vi "WPI_CounterConfigureTimer.vi"(8 "error in (no error)":errorcluster, 9 "Number Samples to Average":u8=1 min=1 max=128, 10 "MaxPeriod (sec)":dbl=0.05, 11 "CounterDevRef in":T1) -> (0 "error out":errorcluster, 3 "CounterDevRef out":T1)   [LabVIEW 2017]
doc: "Configures the timer on the counter. Use this VI to specify the maximum time between pulses that can elapse before the application considers the counter stopped and to specify the number of samples of the timer to average when calculating the period. Use the Get VI to determine whether the counter is stopped.\n\nThis software is licensed. Open the labview\\readme\\WPI Robotics Library Open Source License.txt file for more information."
uses:
  <vilib>/Rock Robotics/WPI/Counter/WPI_CounterDevRef.ctl
  <vilib>/Rock Robotics/SystemInterfaces/Counter/FPGA_CounterCtrSystemIndex.ctl
  <vilib>/Rock Robotics/SystemInterfaces/Counter/FPGA_CounterERRInvalidResource.vi
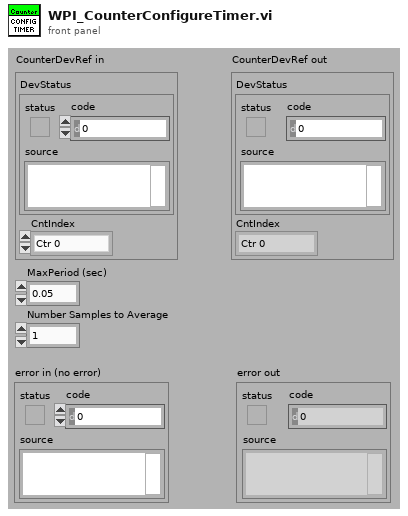
[diagram p1: front panel]
types:
  T1 = typedef "WPI_CounterDevRef.ctl" = cluster{"DevStatus":errorcluster, "CntIndex":T2}
  T2 = typedef "FPGA_CounterCtrSystemIndex.ctl" = enum8{"Ctr 0", "Ctr 1", "Ctr 2", "Ctr 3", "Ctr 4", "Ctr 5", "Ctr 6", "Ctr 7", "Invalid"}
  T3 = typedef "FPGA_CounterCtrDevRef.ctl" = cluster{"DevStatus":errorcluster, "CntIndex":T2}
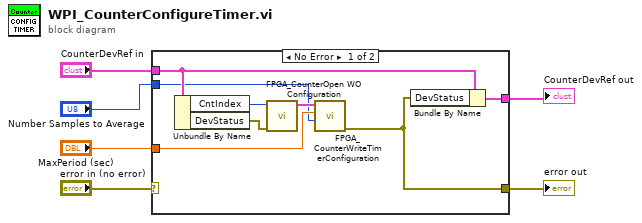
[diagram p0: block diagram]
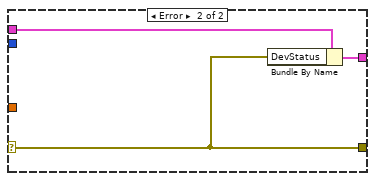
[diagram p2: hidden frame]
diagram:
  n1 = case shown="No Error" "error in (no error)" {
    selector: "error in (no error)" -> [_ w15]
    tunnel: "CounterDevRef in" -> [w14 w17]
    tunnel: [w13 w16] -> w5
    tunnel: [w8 w15] -> w3
    tunnel: "MaxPeriod (sec)" -> [w9 _]
    tunnel: "Number Samples to Average" -> [w7 _]
    frame No Error {
      n2 = Unbundle By Name(w14) -> ("CntIndex"=w11:T2, "DevStatus"=w12:errorcluster)
      n3 = call <vilib>:"FPGA_CounterOpen WO Configuration.vi"("error in"=w12, "CntIndex"=w11) -> ("Ctr Ref"=w10:T3)  [unwired: 1 in, 8 out]
      n4 = call <vilib>:"FPGA_CounterWriteTimerConfiguration.vi"("Average Size"=w7, "StallPeriod (s)"=w9, "Ctr Ref in"=w10) -> ("error out"=w8:errorcluster)  [unwired: 2 in, 6 out]
      n5 = Bundle By Name(cluster=w14, "DevStatus"=w8) -> (w13:T1)
    }
    frame Error {
      n6 = Bundle By Name(cluster=w17, "DevStatus"=w15) -> (w16:T1)
    }
  }
  "CounterDevRef out" <- w5
  "error out" <- w3
